vi "getRampEvent.vi"(8 "error in (no error)":errorcluster, 11 "RampAction in":refnum<class "RampAction.lvclass">) -> (0 "error out":errorcluster, 2 "RampEvent":refnum<class "RampEvent.lvclass">, 3 "RampAction out":refnum<class "RampAction.lvclass">)   [LabVIEW 2011, in "Views.lvlib" / "ScriptEditor.lvlib" / "RampAction.lvclass"]
uses:
  RampAction.lvclass
  Tools/Scripting/ScriptingEvent/ScriptEvents/Ramp/RampEvent/RampEvent.lvclass
  ActionPanel.lvclass
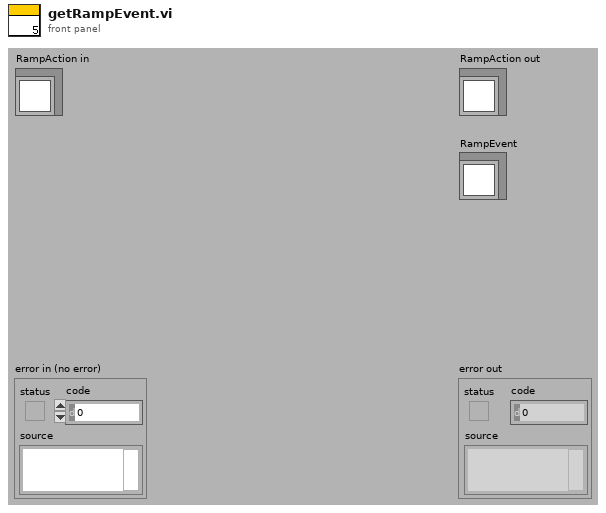
[diagram p1: front panel]
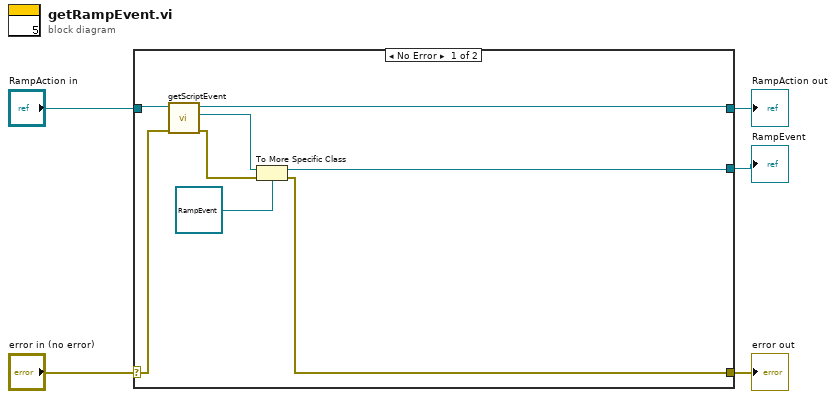
[diagram p0: block diagram]
diagram:
  n1 = case shown="No Error" "error in (no error)" {
    selector: "error in (no error)" -> [w11 w15]
    tunnel: [w6 w15] -> w4
    tunnel: [w12 w14] -> w2
    tunnel: "RampAction in" -> [w13 w14]
    tunnel: [w7 _] -> w1
    frame No Error {
      n2 = call "getScriptEvent.vi"("error in (no error)"=w11, "ActionPanel.lvclass in"=w13) -> ("error out"=w8:errorcluster, "ScriptEvent.lvclass"=w10:refnum<class "ScriptEvent.lvclass">, "ActionPanel.lvclass out"=w12:refnum<class "RampAction.lvclass">)  [unwired: 7 in]
      n3 = To More Specific Class(target class=refnum<class "RampEvent.lvclass"> refnum ("Tools.lvlib:Scripting.lvlib:RampEvent.lvclass"), reference=w10, error in=w8) -> (specific class reference=w7:refnum<class "RampEvent.lvclass">, error out=w6:errorcluster)
    }
    frame Error {
    }
  }
  "error out" <- w4
  "RampAction out" <- w2
  "RampEvent" <- w1
